vi "UpdateHardwareData.vi"(8 "Error In":errorcluster, 10 "Hardware Data Structures":T4, 11 "Hardware Collect Data In":T1) -> (0 "Error Out":errorcluster, 3 "Hardware Collect Data Out":T1)   [LabVIEW 2012]
uses:
  HardwareDataStructures.ctl
  PXI6229Data.ctl
  CurrentMeterData.ctl
  HardwareLogData.ctl
  HardwareDisplayData.ctl
  HardwareCollectData.ctl
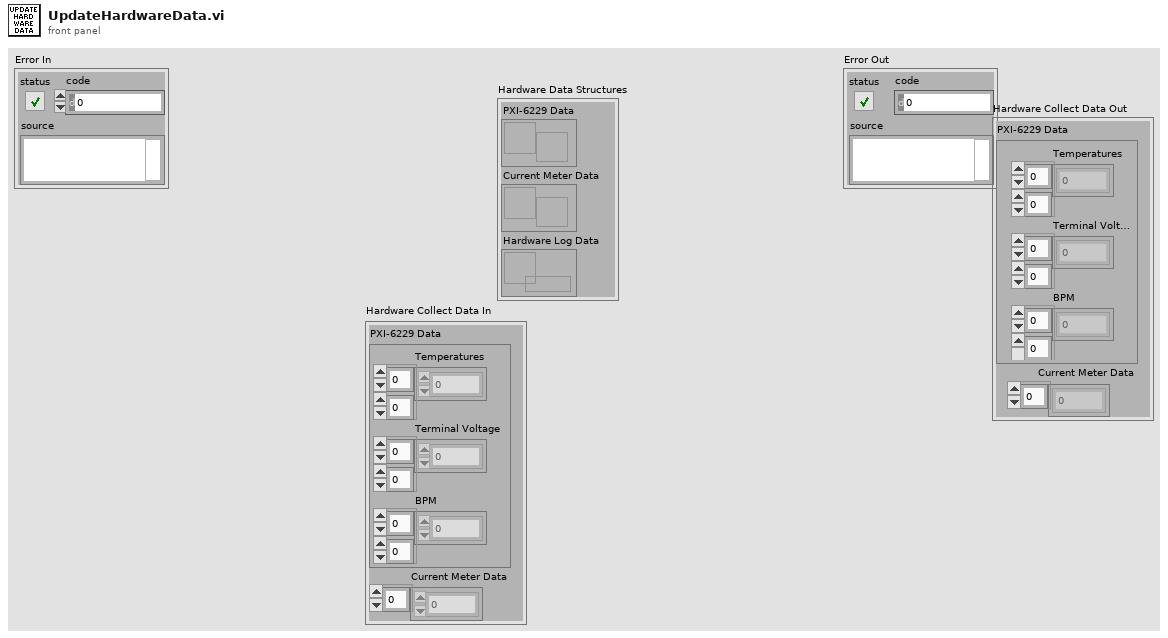
[diagram p1: front panel]
types:
  T1 = typedef "HardwareCollectData.ctl" = cluster{"PXI-6229 Data":T2, "Current Meter Data":T3}
  T2 = typedef "PXI6229Data.ctl" = cluster{"Temperatures":dbl[][], "Terminal Voltage":dbl[][], "BPM":dbl[][]}
  T3 = typedef "CurrentMeterData.ctl" = dbl[]
  T4 = typedef "HardwareDataStructures.ctl" = cluster{"PXI-6229 Data":refnum<notifier>, "Current Meter Data":refnum<notifier>, "Hardware Log Data":refnum<queue>}
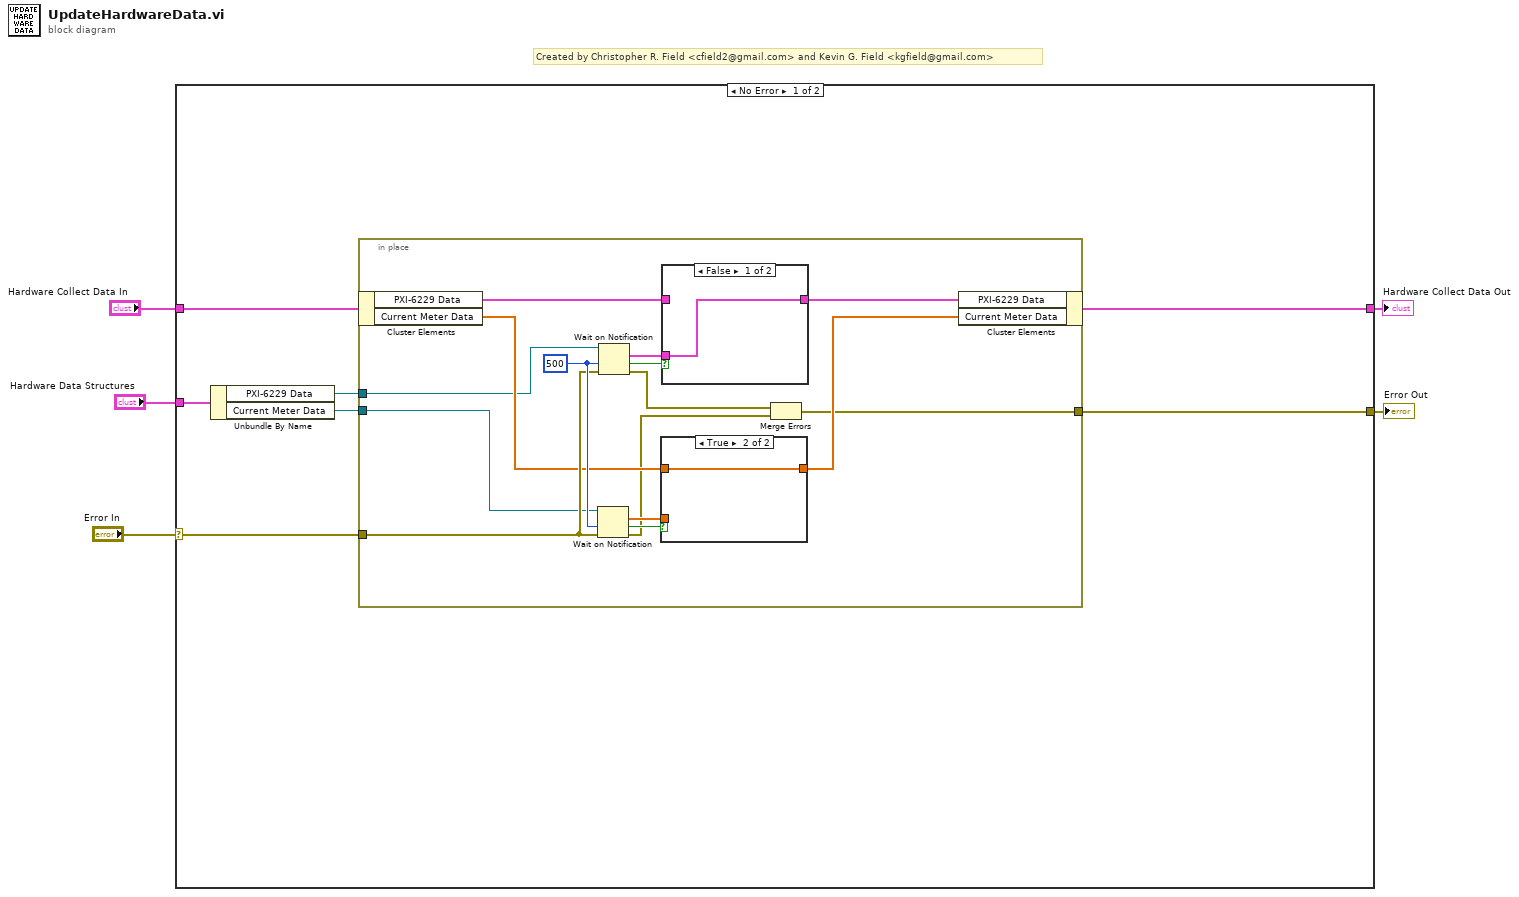
[diagram p0: block diagram]
diagram:
  # "Created by Christopher R. Field <cfield2@gmail.com> and Kevin G. Field <kgfield@gmail.com>"
  n1 = case shown="No Error" "Error In" {
    selector: "Error In" -> [w11 w32]
    tunnel: "Hardware Collect Data In" -> [w12 w33]
    tunnel: [w10 w32] -> w3
    tunnel: [w9 w33] -> w2
    tunnel: "Hardware Data Structures" -> [w8 _]
    frame No Error {
      n2 = Unbundle By Name(w8) -> ("PXI-6229 Data"=w7:refnum<notifier>, "Current Meter Data"=w6:refnum<notifier>)
      n3 = in-place {
        in-place-border: w11 -> [w22]
        in-place-border: [w15] -> w10
        in-place-border: w7 -> [w14]
        in-place-border: w6 -> [w13]
        w27 = 500 ("timeout in ms (-1)")
        n4 = in-place-cluster #1(w12) -> ("PXI-6229 Data"=w21:T2, "Current Meter Data"=w19:T3)
        n5 = Wait on Notification(notifier=w13, timeout in ms (-1)=w27, error in (no error)=w22) -> (notification=w23:T3, timed out?=w24:bool, error out=w16:errorcluster)  [unwired: 1 in, 1 out]
        n6 = Wait on Notification(notifier=w14, timeout in ms (-1)=w27, error in (no error)=w22) -> (notification=w25:T2, timed out?=w26:bool, error out=w17:errorcluster)  [unwired: 1 in, 1 out]
        n7 = case shown="True" w24 {
          tunnel: w23 -> [w28 _]
          tunnel: [w28 w29] -> w18
          tunnel: w19 -> [_ w29]
          frame False {
          }
          frame True {
          }
        }
        n8 = case shown="False" w26 {
          tunnel: w25 -> [w30 _]
          tunnel: [w30 w31] -> w20
          tunnel: w21 -> [_ w31]
          frame False {
          }
          frame True {
          }
        }
        n9 = Merge Errors(w17, w16) -> (w15:errorcluster)
        n10 = in-place-cluster #1("PXI-6229 Data"=w20, "Current Meter Data"=w18) -> (w9:T1)
      }
    }
    frame Error {
    }
  }
  "Error Out" <- w3
  "Hardware Collect Data Out" <- w2
